vi "Copy .LLB to NI VeriStand dir.vi"(5 "Files Generated by Build":path[](array[path]), 6 "Top Level/Always Included VIs":path[](array[path]), 7 "Destination Path":path, 8 "error in (no error)":errorcluster, 9 "Target Name":string, 10 "Build Specification Name":string, 11 "Project Path":path) -> (0 "error out":errorcluster)   [LabVIEW 2015]
doc: "This VI is called after each run of a build specification. The VI will copy the generated LLB (Engine or System Explorer) into the VeriStand Custom Device folder (...\\Documents\\National Instruments\\NI VeriStand 2013...)."
uses:
  <vilib>/Utility/sysdir.llb/System Directory Type.ctl
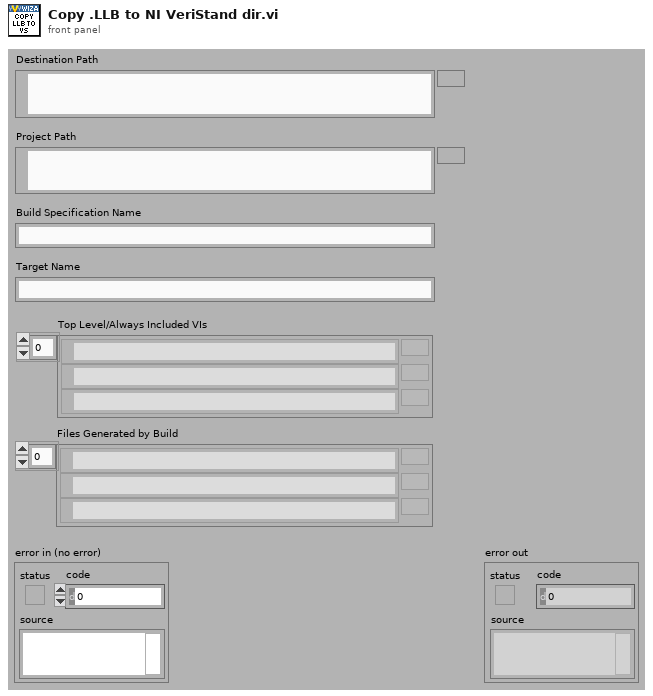
[diagram p1: front panel]
types:
  T1 = typedef "System Directory Type.ctl" = i32
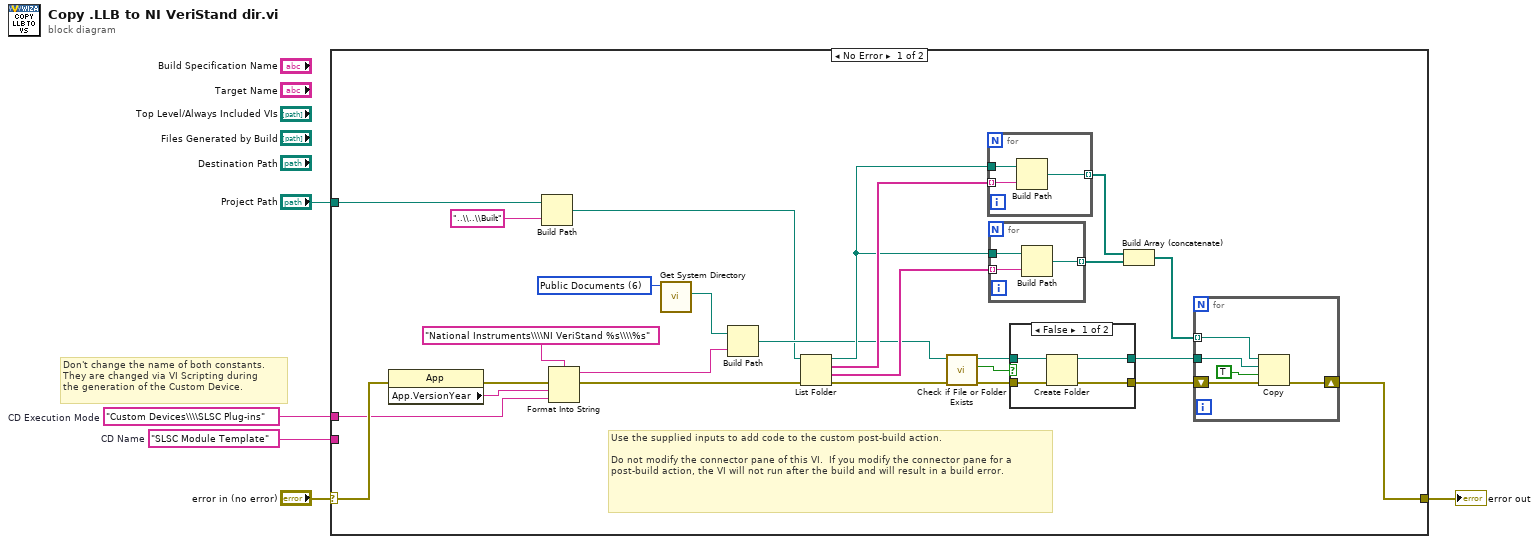
[diagram p0: block diagram]
diagram:
  w1 = "SLSC Module Template"  # CD Name
  w2 = "Custom Devices\\\\SLSC Plug-ins"  # CD Execution Mode
  # "Don't change the name of both constants.\nThey are changed via VI Scripting during\nthe generation of the Custom Device."
  n1 = case shown="No Error" "error in (no error)" {
    selector: "error in (no error)" -> [w14 w49]
    tunnel: [w16 w49] -> w3
    tunnel: "Project Path" -> [w11 _]
    tunnel: w2 -> [w7 _]
    tunnel: w1 -> [_ _]
    frame No Error {
      w19 = T1 6 items=["User Home"=0, "User Desktop"=1, "User Documents"=2, "User Application Data"=3, "User Preferences"=4, "User Temporary"=5, "Public Documents"=6, "Public Application Data"=7, "Public Preferences"=8, "Public Cache"=13, "System Core Libraries"=9, "System Installed Libraries"=10, "Application Files"=11, "Boot Volume Root"=12] ("system directory type")
      # "Use the supplied inputs to add code to the custom post-build action.\n\nDo not modify the connector pane of this VI.  If you modify the connector pane for a post-build action, the VI will not run after the build and will result in a build error."
      n2 = property class="App"(error in=w14) -> (error out=w18:errorcluster, "App.VersionYear"=w17:string)  [unwired: 1 in, 1 out]
      n3 = Build Path(base path=w11, name or relative path="..\\..\\Built") -> (appended path=w8:path)
      n4 = Format Into String(format string="National Instruments\\\\NI VeriStand %s\\\\%s" ("name or relative path"), error in=w18, w17, w7) -> (resulting string=w21:string, error out=w13:errorcluster)  [unwired: 1 in]
      n5 = call <vilib>:"Get System Directory.vi"("system directory type"=w19) -> ("system directory"=w20:path)  [unwired: 10 in]
      n6 = Build Path(base path=w20, name or relative path=w21) -> (appended path=w15:path)
      n7 = List Folder(path=w8, error in=w13) -> (path out=w24:path, filenames=w31:string[], folder names=w25:string[], error out=w22:errorcluster)  [unwired: 2 in]
      n8 = call <vilib>:"Check if File or Folder Exists.vi"("error in (no error)"=w22, "path"=w15) -> ("error out"=w26:errorcluster, "file or folder exists?"=w28:bool, "dup path"=w27:path)  [unwired: 7 in]
      n9 = for {
        tunnel: w31 -> [w47] mode=indexing
        tunnel: w24 -> [w48]
        tunnel: [w46] -> w30 mode=indexing
        n10 = Build Path(base path=w48, name or relative path=w47) -> (appended path=w46:path)
      }
      n11 = for {
        tunnel: w25 -> [w44] mode=indexing
        tunnel: w24 -> [w45]
        tunnel: [w43] -> w23 mode=indexing
        n12 = Build Path(base path=w45, name or relative path=w44) -> (appended path=w43:path)
      }
      n13 = case shown="False" w28 {
        tunnel: w27 -> [w35 w37]
        tunnel: w26 -> [w34 w36]
        tunnel: [w33 w37] -> w10
        tunnel: [w32 w36] -> w9
        frame False {
          n14 = Create Folder(path (use dialog)=w35, error in=w34) -> (created path=w33:path, error out=w32:errorcluster)  [unwired: 1 in, 1 out]
        }
        frame True {
        }
      }
      n15 = Build Array (concatenate)(w30, w23) -> (w29:path[])
      n16 = for {
        tunnel: w29 -> [w39] mode=indexing
        shift-right: [w40] -> w16
        shift-left: w9 -> [w41]
        tunnel: w10 -> [w38]
        n17 = Copy(8:w41, 9:TRUE ("overwrite (F)"), 10:w38, 11:w39) -> (0:w40:errorcluster)  [unwired: 1 in, 2 out]
      }
    }
    frame Error {
    }
  }
  "error out" <- w3
